vi "Terminal Wire Joints.vi"(10 "Is Source?":bool, 11 "Joints":T1(array[cluster])) -> (2 "Horizontal Position":i16, 3 "Vertical Position":i16)   [LabVIEW 2019, in "Builtins.lvlib"]
doc: "Find the adjacent wire terminal position.\n\nCreated by: Ryan Pacini"
uses:
  Builtins.lvlib
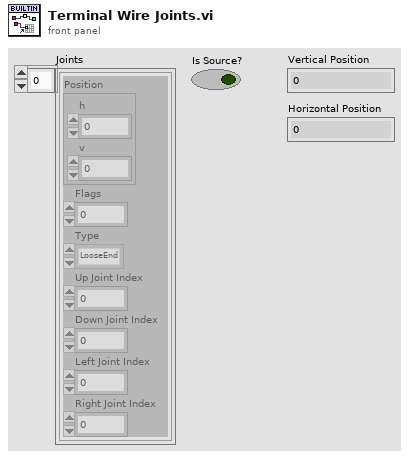
[diagram p1: front panel]
types:
  T1 = cluster{"Position":cluster{"h":i16, "v":i16}, "Flags":i32, "Type":enum32{"LooseEnd", "Endpoint", "Bend", "Junction"}, "Up Joint Index":i16, "Down Joint Index":i16, "Left Joint Index":i16, "Right Joint Index":i16}[]
  T2 = enum32{"LooseEnd", "Endpoint", "Bend", "Junction"}
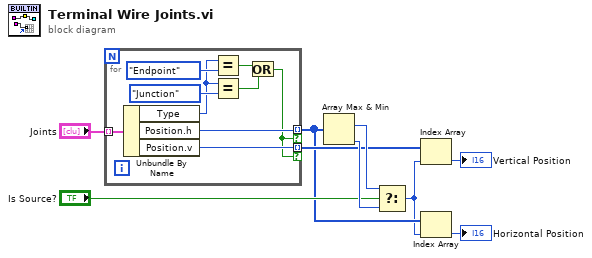
[diagram p0: block diagram]
diagram:
  n1 = for {
    tunnel: "Joints" -> [w18] mode=indexing
    tunnel: [w12] -> w3 mode=indexing if=w10
    tunnel: [w11] -> w7 mode=indexing if=w10
    n2 = Unbundle By Name(w18) -> ("Type"=w15:T2, "Position.h"=w12:i16, "Position.v"=w11:i16)
    n3 = Equal?(x=w15, y=T2."Endpoint" ("Type")) -> (x = y?=w14:bool)
    n4 = Equal?(x=w15, y=T2."Junction" ("Type")) -> (x = y?=w13:bool)
    n5 = Or(x=w14, y=w13) -> (x .or. y?=w10:bool)
  }
  n6 = Array Max & Min(array=w3) -> (max index (indices)=w8:i32, min index (indices)=w9:i32)  [unwired: 2 out]
  n7 = Select(t=w8, s="Is Source?", f=w9) -> (s? t:f=w2:i32)
  n8 = Index Array(array=w7, index=w2) -> (element=→"Vertical Position":i16)
  n9 = Index Array(array=w3, index=w2) -> (element=→"Horizontal Position":i16)
